vi "Set Update Event.vi"(8 "error in (no error)":errorcluster, 10 "App Update Event":refnum<user-event>, 11 "App Watcher in":refnum<class "App Watcher.lvclass">) -> (0 "error out":errorcluster, 3 "App Watcher out":refnum<class "App Watcher.lvclass">)   [LabVIEW 2020, in "PicoG-App.lvlib" / "App Watcher.lvclass"]
uses:
  App Watcher.lvclass
  App Update Data.ctl
  ViaApp/ViaApp.lvclass
  App Watcher.lvclass/App Watcher.ctl
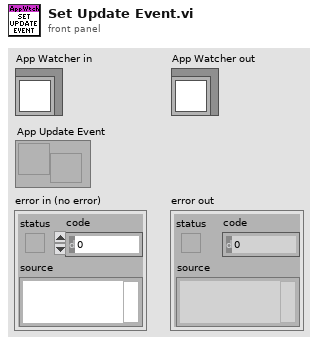
[diagram p1: front panel]
types:
  T1 = typedef "PicoG-App.lvlib/App Watcher.lvclass/Ref Data.ctl" = cluster{"App Map":map{path, refnum<class "ViaApp.lvclass">}, "App Update Event":refnum<user-event>}
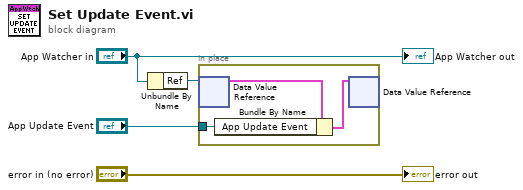
[diagram p0: block diagram]
diagram:
  n1 = Unbundle By Name("App Watcher in") -> ("Ref"=w3:refnum<data-value>)
  n2 = in-place {
    in-place-border: "App Update Event" -> [w5]
    n3 = in-place-dvr #1(w3) -> (w7:T1)  [unwired: 1 out]
    n4 = Bundle By Name(cluster=w7, "App Update Event"=w5) -> (w6:T1)
    n5 = in-place-dvr #1(w6) -> ()  [unwired: 2 out]
  }
  "error out" <- "error in (no error)"
  "App Watcher out" <- "App Watcher in"
